vi "pulsed ODMR.vi"() -> ()   [LabVIEW 2012]
uses:
  <vilib>/DAQmx/read.llb/DAQmx Read (Counter U32 1Chan 1Samp).vi
  <vilib>/Utility/file.llb/Write To Spreadsheet File (DBL).vi
  <vilib>/DAQmx/miscellaneous.llb/DAQmx Fill In Error Info.vi
  <vilib>/DAQmx/create/channels.llb/DAQmx Create Channel (CI-Count Edges).vi
  <vilib>/DAQmx/create/channels.llb/DAQmx Create Channel (CO-Pulse Generation-Ticks).vi
  <vilib>/DAQmx/configure/timing.llb/DAQmx Timing (Implicit).vi
  <vilib>/DAQmx/configure/timing.llb/DAQmx Timing (Sample Clock).vi
  <resource>/objmgr/daqmx.rc
panel:
  out "Scan":i32=1
  in  "N Scans":i32=200
  out "freq":dbl=3169000000.0
  out "diff":dbl=864.0
  out "loop":i32=169
  in  "file path (dialog if empty)":path=path "C:/Users/Ouyang Group/Documents/Data/10-10-16/MNP 4 on CPW 5mW x157 y142 B0.4V pulsed ODMR sweep 2"
  out "Z Position 2":dbl=37.2
  out "Y Position 2":dbl=132.5360878371843
  out "X Position 2":dbl=154.08405055143967
  in  "CW for tracking":bool
  in  "Y Parameters":T1={"Number of Y Steps"=200, "Max Y (V)"=2.0, "Min Y (V)"=-2.0}
  in  "X":T2={"Number of X Steps"=200, "Max X (V)"=2.0, "Min X (V)"=-2.0}
  in  "Z Position":dbl=37.2
  in  "Y Position":dbl=132.0
  in  "X Position":dbl=154.0
  in  "Z-track?":bool=TRUE
  out "XY Graph":cluster{"Y":dbl[], "Y":dbl[]}[](graph)=[{"Y"=[3000000000.0, 3001000000.0, 3002000000.0, 3003000000.0, 3004000000.0, 3005000000.0, 3006000000.0, 3007000000.0, 3008000000.0, 3009000000.0, 3010000000.0, 3011000000.0, 3012000000.0, 3013000000.0, 3014000000.0, 3015000000.0, 3016000000.0, 3017000000.0, 3018000000.0, 3019000000.0, 3020000000.0, 3021000000.0, 3022000000.0, 3023000000.0, 3024000000.0, 3025000000.0, 3026000000.0, 3027000000.0, 3028000000.0, 3029000000.0, 3030000000.0, 3031000000.0, 3032000000.0, 3033000000.0, 3034000000.0, 3035000000.0, 3036000000.0, 3037000000.0, 3038000000.0, 3039000000.0, 3040000000.0, 3041000000.0, 3042000000.0, 3043000000.0, 3044000000.0, 3045000000.0, 3046000000.0, 3047000000.0, 3048000000.0, 3049000000.0, 3050000000.0, 3051000000.0, 3052000000.0, 3053000000.0, 3054000000.0, 3055000000.0, 3056000000.0, 3057000000.0, 3058000000.0, 3059000000.0, 3060000000.0, 3061000000.0, 3062000000.0, 3063000000.0, 3064000000.0, 3065000000.0, 3066000000.0, 3067000000.0, 3068000000.0, 3069000000.0, 3070000000.0, 3071000000.0, 3072000000.0, 3073000000.0, 3074000000.0, 3075000000.0, 3076000000.0, 3077000000.0, 3078000000.0, 3079000000.0, 3080000000.0, 3081000000.0, 3082000000.0, 3083000000.0, 3084000000.0, 3085000000.0, 3086000000.0, 3087000000.0, 3088000000.0, 3089000000.0, 3090000000.0, 3091000000.0, 3092000000.0, 3093000000.0, 3094000000.0, 3095000000.0, 3096000000.0, 3097000000.0, 3098000000.0, 3099000000.0, 3100000000.0, 3101000000.0, 3102000000.0, 3103000000.0, 3104000000.0, 3105000000.0, 3106000000.0, 3107000000.0, 3108000000.0, 3109000000.0, 3110000000.0, 3111000000.0, 3112000000.0, 3113000000.0, 3114000000.0, 3115000000.0, 3116000000.0, 3117000000.0, 3118000000.0, 3119000000.0, 3120000000.0, 3121000000.0, 3122000000.0, 3123000000.0, 3124000000.0, 3125000000.0, 3126000000.0, 3127000000.0, 3128000000.0, 3129000000.0, 3130000000.0, 3131000000.0, 3132000000.0, 3133000000.0, 3134000000.0, 3135000000.0, 3136000000.0, 3137000000.0, 3138000000.0, 3139000000.0, 3140000000.0, 3141000000.0, 3142000000.0, 3143000000.0, 3144000000.0, 3145000000.0, 3146000000.0, 3147000000.0, 3148000000.0, 3149000000.0, 3150000000.0, 3151000000.0, 3152000000.0, 3153000000.0, 3154000000.0, 3155000000.0, 3156000000.0, 3157000000.0, 3158000000.0, 3159000000.0, 3160000000.0, 3161000000.0, 3162000000.0, 3163000000.0, 3164000000.0, 3165000000.0, 3166000000.0, 3167000000.0, 3168000000.0, 3169000000.0], "Y"=[20897.0, 22852.0, 22779.0, 22894.0, 22927.0, 22741.0, 22573.0, 22733.0, 22830.0, 22883.0, 22762.0, 22899.0, 22761.0, 22773.0, 22842.0, 22907.0, 22850.0, 22605.0, 22781.0, 22681.0, 22700.0, 22960.0, 23015.0, 22551.0, 22696.0, 22371.0, 22868.0, 22865.0, 22767.0, 22787.0, 22656.0, 22872.0, 22848.0, 22750.0, 22901.0, 22775.0, 22816.0, 21819.0, 22361.0, 22464.0, 22800.0, 22880.0, 22472.0, 22759.0, 22543.0, 22595.0, 23074.0, 22794.0, 22857.0, 22851.0, 22603.0, 22581.0, 22045.0, 22687.0, 22517.0, 22600.0, 22685.0, 22887.0, 22876.0, 22789.0, 22503.0, 22751.0, 22684.0, 22564.0, 22897.0, 22744.0, 21980.0, 22771.0, 22841.0, 22311.0, 22234.0, 22304.0, 22403.0, 22585.0, 22374.0, 22604.0, 22287.0, 22575.0, 22599.0, 22689.0, 22662.0, 22060.0, 22437.0, 22293.0, 21954.0, 21800.0, 21174.0, 20810.0, 20547.0, 20230.0, 20049.0, 19600.0, 19389.0, 18817.0, 18827.0, 18800.0, 18771.0, 19210.0, 19068.0, 19533.0, 19442.0, 19668.0, 19746.0, 20480.0, 21116.0, 21287.0, 21615.0, 21711.0, 21860.0, 22239.0, 22301.0, 22345.0, 22646.0, 22502.0, 22803.0, 22744.0, 22476.0, 22049.0, 22378.0, 22415.0, 22489.0, 22623.0, 22255.0, 22383.0, 22791.0, 22426.0, 22564.0, 22666.0, 22587.0, 22692.0, 22619.0, 22746.0, 22870.0, 22967.0, 22739.0, 23010.0, 22733.0, 22399.0, 22777.0, 22571.0, 22573.0, 22914.0, 22383.0, 23082.0, 22534.0, 22649.0, 22510.0, 22903.0, 22967.0, 22609.0, 22872.0, 22608.0, 22798.0, 22757.0, 22774.0, 22548.0, 22722.0, 22710.0, 22449.0, 22814.0, 22959.0, 22831.0, 22570.0, 22918.0, 23017.0, 22810.0, 22802.0, 22761.0, 22627.0, 22371.0]}]
  in  "Freq Max":dbl=3120000000.0
  in  "Freq  Step":dbl=250000000.0
  in  "Freq Min":dbl=3060000000.0
  in  "power":dbl=-9.0
  in  "stop":bool
  in  "Path to spinapi.dll":path=path "C:/SpinCore/SpinAPI/dll/spinapi64.dll"
  in  "Pulse offset":dbl
  in  "Rabi Freq":dbl=8895000.0
  in  "MW Delay":dbl=2e-08
  in  "APD signal width":dbl=3e-07
  in  "Signal Delay":dbl=7.6e-07
  in  "AOM Rest time":dbl=1e-06
  in  "AOM Pulse length":dbl=2.5e-06
  in  "N Loop":i32=100000
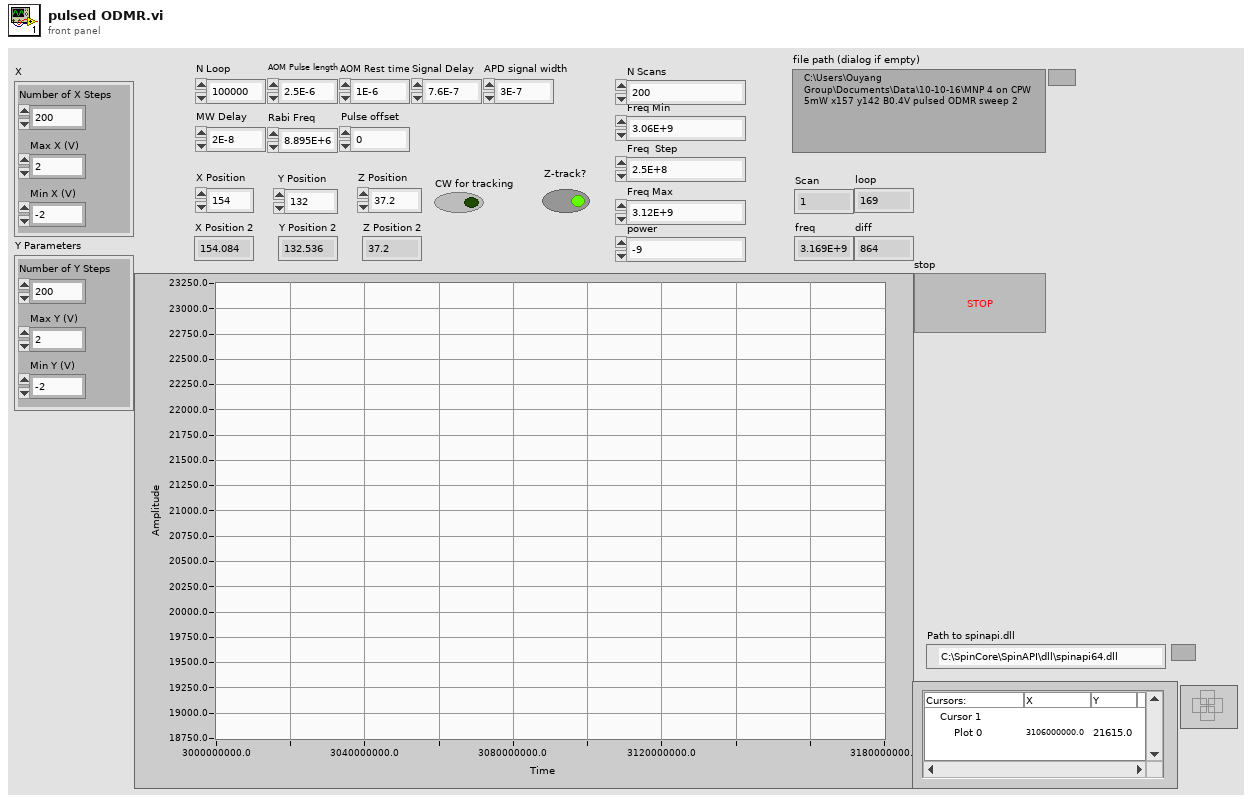
[diagram p1: front panel]
types:
  T1 = cluster{"Number of Y Steps":i32, "Max Y (V)":dbl, "Min Y (V)":dbl}
  T2 = cluster{"Number of X Steps":i32, "Max X (V)":dbl, "Min X (V)":dbl}
  T3 = enum16{"Pulse Program", "Frequency Registers", "TX Phase Registers", "RX Phase Registers"}
  T4 = cluster{"Instruct Data":i32, "Op Code":i32, "Flags":bool[], "Comments":string, "Time (s)":dbl}[]
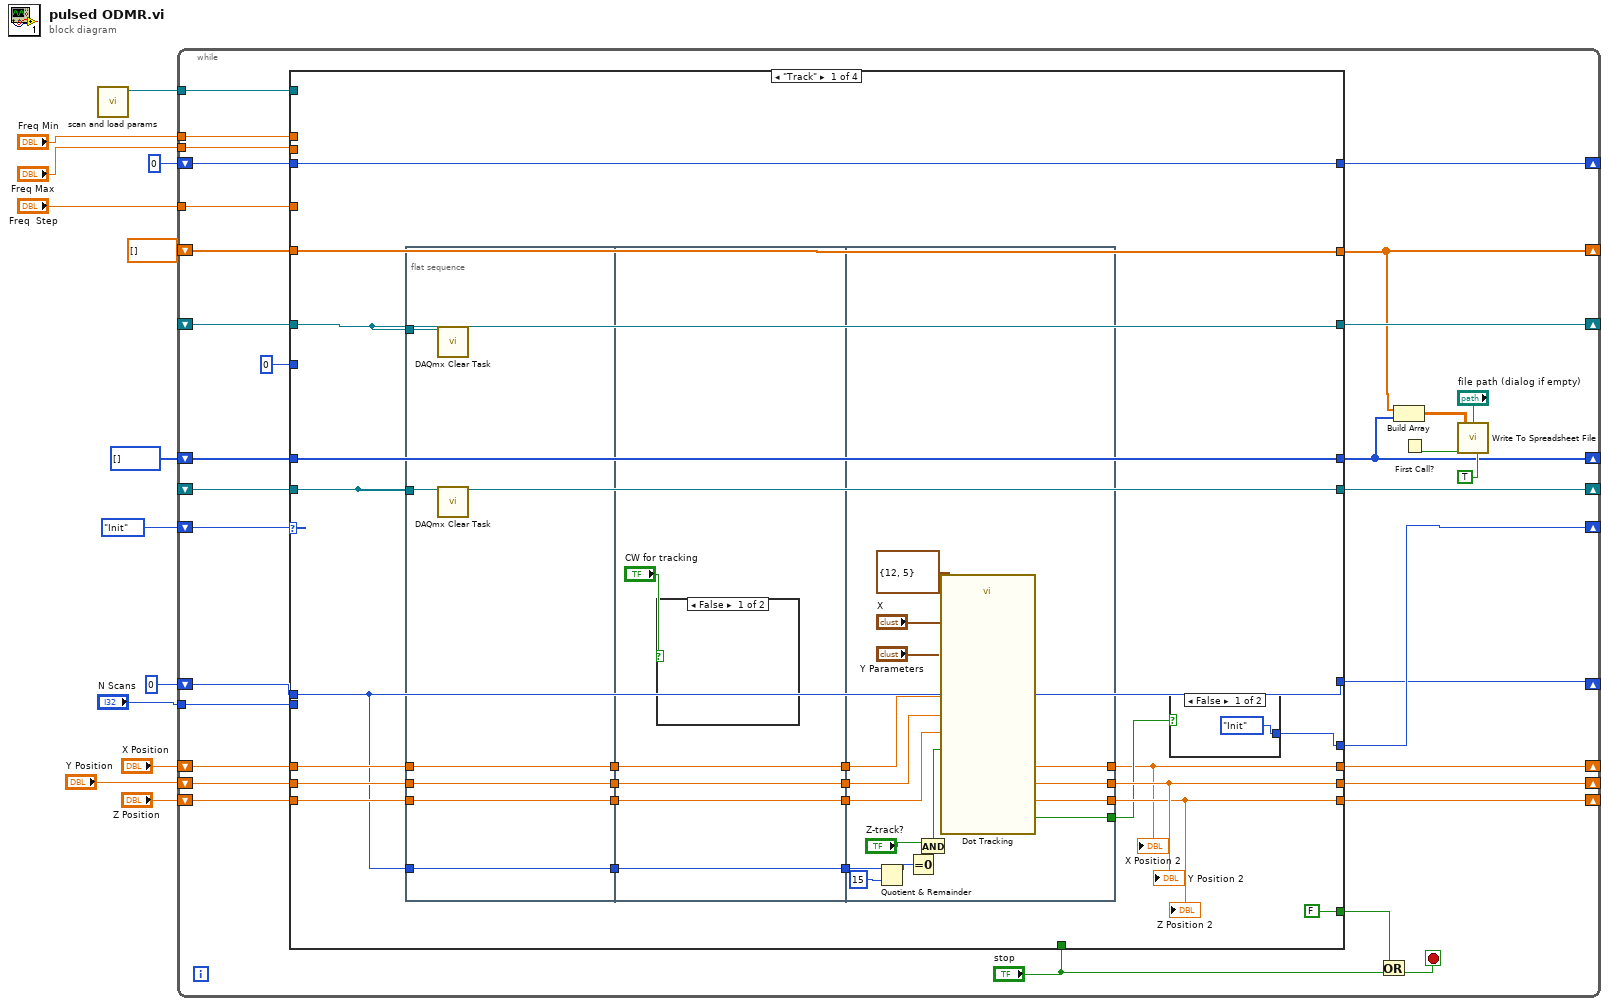
[diagram p0: block diagram]
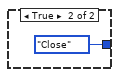
[diagram p2: hidden frame]
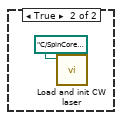
[diagram p3: hidden frame]
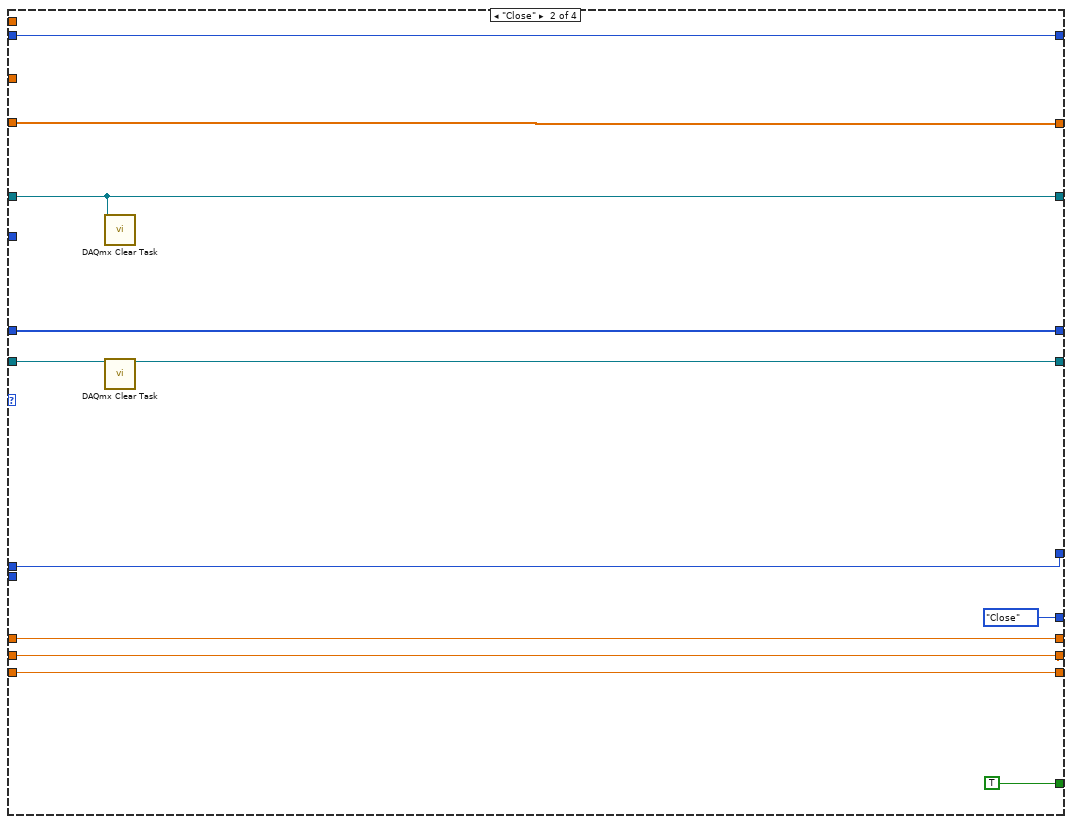
[diagram p4: hidden frame]
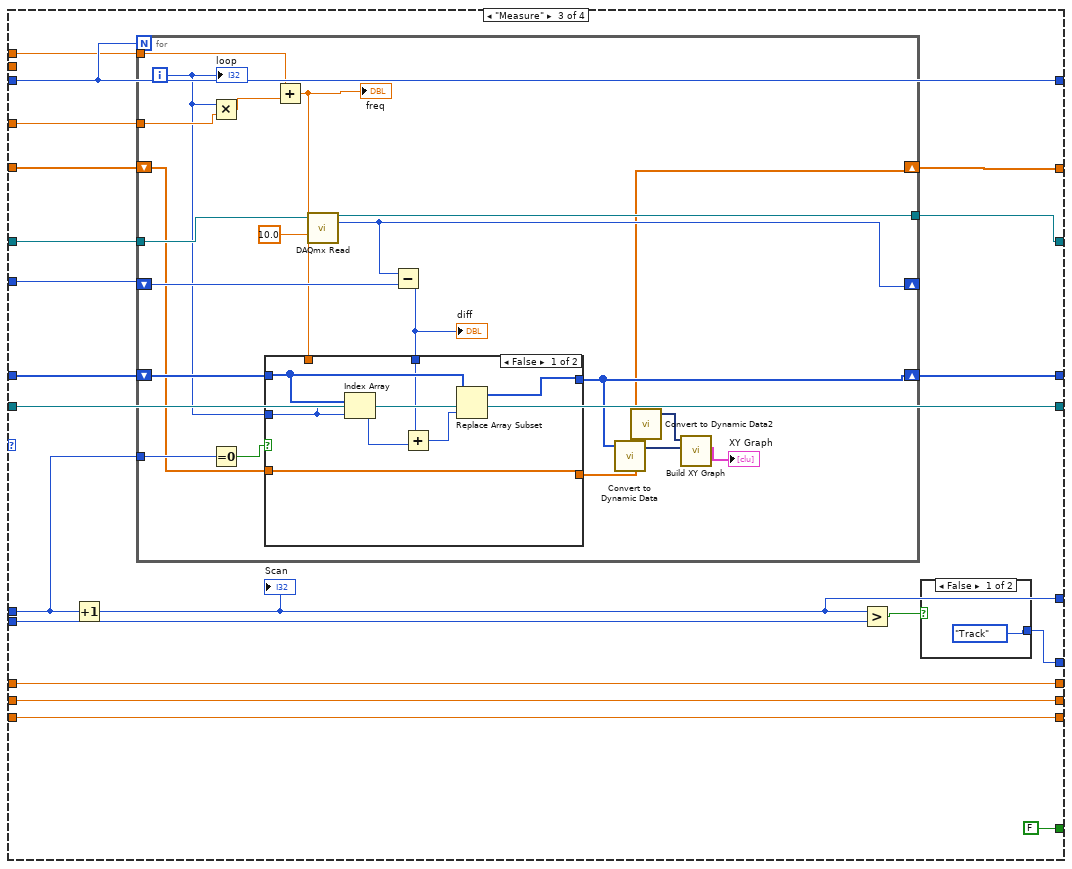
[diagram p5: hidden frame]
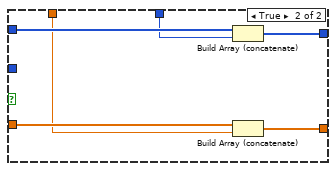
[diagram p6: hidden frame]
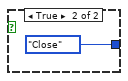
[diagram p7: hidden frame]
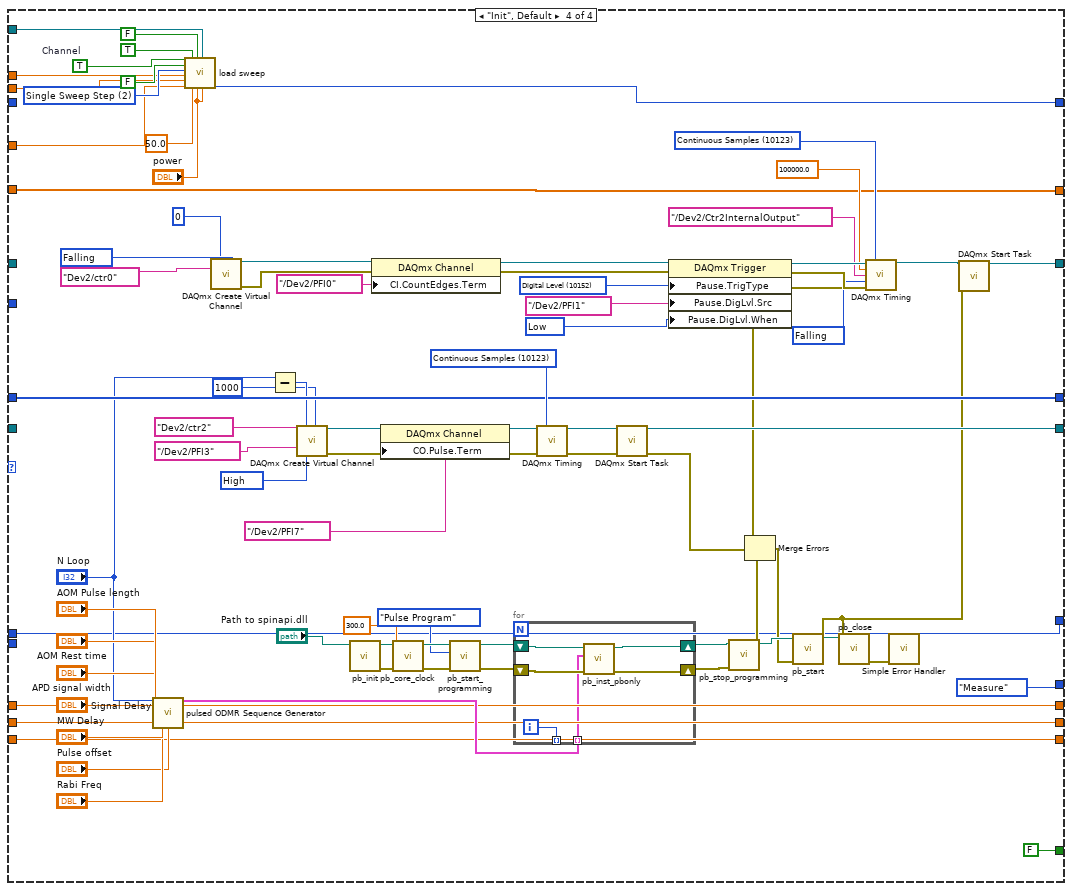
[diagram p8: hidden frame]
diagram:
  n1 = call "scan and load params.vi"() -> ("Serial Port Select"=w7:refnum<visa-resource-name>)  [unwired: 9 out]
  n2 = while {
    shift-right: [w40] -> _
    shift-left: enum16{"Init", "Track", "Measure", "Close", ""}."Init" -> [w46]
    shift-right: [w45] -> _
    shift-left: _ -> [w33]
    shift-right: [w44] -> _
    shift-left: _ -> [w34]
    shift-right: [w15] -> _
    shift-left: u32[] [] -> [w42]
    shift-right: [w28] -> _
    shift-left: dbl[] [] -> [w41]
    shift-right: [w39] -> _
    shift-left: "X Position" -> [w30]
    shift-right: [w38] -> _
    shift-left: "Y Position" -> [w36]
    shift-right: [w37] -> _
    shift-left: "Z Position" -> [w35]
    tunnel: w7 -> [w23]
    tunnel: "Freq  Step" -> [w20]
    tunnel: "Freq Max" -> [w21]
    tunnel: "Freq Min" -> [w22]
    shift-right: [w19] -> _
    shift-left: u16 0 ("Number\nof Points") -> [w18]
    tunnel: "N Scans" -> [w17]
    shift-right: [w14] -> _
    shift-left: 0 -> [w16]
    stop <- w32 stop-if-true
    n3 = case shown="\"Track\"" w46 {
      tunnel: [w53 w110 w124 w195] -> w45
      tunnel: [w52 w109 w117 w194] -> w44
      tunnel: "stop" -> [_ _ _ _]
      tunnel: w42 -> [w62 w108 w130 w192]
      tunnel: w41 -> [w57 w103 w129 w188]
      tunnel: [w62 w108 w128 w192] -> w15
      tunnel: [w57 w103 w121 w188] -> w28
      tunnel: [w61 enum16{"Init", "Track", "Measure", "Close", ""}."Close" w127 enum16{"Init", "Track", "Measure", "Close", ""}."Measure"] -> w40
      tunnel: [w50 w102 w120 w187] -> w39
      tunnel: [w69 w107 w123 w190] -> w38
      tunnel: [w68 w106 w122 w189] -> w37
      tunnel: w36 -> [w65 w107 w123 w190]
      tunnel: w35 -> [w63 w106 w122 w189]
      tunnel: w34 -> [w52 w109 w125 _]
      tunnel: w33 -> [w53 w110 w124 _]
      tunnel: [FALSE TRUE FALSE FALSE] -> w31
      tunnel: w30 -> [w58 w102 w120 w187]
      tunnel: u32 0 ("data") -> [_ _ w119 _]
      tunnel: w23 -> [_ _ _ w180]
      tunnel: w22 -> [_ _ w116 w172]
      tunnel: w21 -> [_ _ _ w171]
      tunnel: w20 -> [_ _ w115 w170]
      tunnel: [w51 w101 w118 w169] -> w19
      tunnel: w18 -> [w51 w101 w118 _]
      tunnel: w17 -> [_ _ w113 _]
      tunnel: w16 -> [w47 w100 w111 w168]
      tunnel: [w47 w100 w112 w168] -> w14
      frame "Track" {
        n4 = flat-sequence {
          tunnel: w63 -> [w75]
          tunnel: w65 -> [w76]
          tunnel: w58 -> [w77]
          tunnel: [w77] -> w56
          tunnel: [w76] -> w55
          tunnel: [w75] -> w54
          tunnel: w53 -> [w74]
          tunnel: w52 -> [w73]
          tunnel: [w72] -> w48
          tunnel: w47 -> [w72]
          tunnel: [w82] -> w67
          tunnel: [w81] -> w66
          tunnel: [w80] -> w64
          tunnel: w56 -> [w82]
          tunnel: w55 -> [w81]
          tunnel: w54 -> [w80]
          tunnel: [w78] -> w49
          tunnel: w48 -> [w78]
          tunnel: [w99] -> w50
          tunnel: [w98] -> w69
          tunnel: [w97] -> w68
          tunnel: w67 -> [w96]
          tunnel: w66 -> [w95]
          tunnel: w64 -> [w94]
          tunnel: [w90] -> w60
          tunnel: w49 -> [w84]
          frame #0 {
            n5 = call <vilib>:"DAQmx Clear Task.vi"("task in"=w73) -> ()  [unwired: 14 in, 1 out]
            n6 = call <vilib>:"DAQmx Clear Task.vi"("task in"=w74) -> ()  [unwired: 14 in, 1 out]
          }
          frame #1 {
            n7 = case shown="False" "CW for tracking" {
              frame False {
              }
              frame True {
                n8 = call "Load and init CW laser.vi"("path in"=path "C:/SpinCore/SpinAPI/dll/spinapi64.dll") -> ()  [unwired: 11 in]
              }
            }
          }
          frame #2 {
            n9 = Quotient & Remainder(x=w84, y=15) -> (x-y*floor(x/y)=w88:i32)  [unwired: 1 out]
            n10 = Equal To 0?(x=w88) -> (x = 0?=w87:bool)
            n11 = And(x="Z-track?", y=w87) -> (x .and. y?=w85:bool)
            n12 = call "Dot Tracking.vi"("X"="X", "Y Parameters"="Y Parameters", "RS232 settings"=cluster{"Portnumber":i32, "Baudrate":u16} {"Portnumber"=12, "Baudrate"=5}, "X Pos"=w96, "Y pos"=w95, "Z Pos"=w94, "Z-track?"=w85) -> ("X Position"=w99:dbl, "Y Position"=w98:dbl, "Z Position"=w97:dbl, "Gave up?"=w90:bool)  [unwired: 2 in, 3 out]
          }
        }
        n13 = case shown="False" w60 {
          tunnel: [enum16{"Init", "Track", "Measure", "Close", ""}."Init" enum16{"Init", "Track", "Measure", "Close", ""}."Close"] -> w61
          frame False {
          }
          frame True {
          }
        }
        "X Position 2" <- w50
        "Y Position 2" <- w69
        "Z Position 2" <- w68
      }
      frame "Close" {
        n14 = call <vilib>:"DAQmx Clear Task.vi"("task in"=w109) -> ()  [unwired: 14 in, 1 out]
        n15 = call <vilib>:"DAQmx Clear Task.vi"("task in"=w110) -> ()  [unwired: 14 in, 1 out]
      }
      frame "Measure" {
        n16 = Increment(x=w111) -> (x+1=w112:i32)
        "Scan" <- w112
        n17 = for {
          N: w118 -> [_]
          shift-right: [w141] -> w128
          shift-left: w130 -> [w142]
          shift-right: [w132] -> w121
          shift-left: w129 -> [w133]
          tunnel: w125 -> [w149]
          shift-right: [w144] -> _
          shift-left: w119 -> [w146]
          tunnel: [w145] -> w117
          tunnel: w116 -> [w140]
          tunnel: w115 -> [w139]
          tunnel: w111 -> [w136]
          i -> [w134]
          n18 = Multiply(x=w134, y=w139) -> (x*y=w138:dbl)
          n19 = Equal To 0?(x=w136) -> (x = 0?=w135:bool)
          n20 = Add(x=w140, y=w138) -> (x+y=w131:dbl)
          "freq" <- w131
          n21 = call-poly <vilib>:"DAQmx Read.vi"("task/channels in"=w149, "timeout"=10.0) -> ("task out"=w145:refnum<k21>, "data"=w144:u32)  [unwired: 11 in, 1 out]
          n22 = Subtract(x=w144, y=w146) -> (x-y=w137:u32)
          "diff" <- w137
          n23 = case shown="False" w135 {
            tunnel: w142 -> [w157 w163]
            tunnel: [w152 w162] -> w141
            tunnel: w137 -> [w154 w161]
            tunnel: w134 -> [w156 _]
            tunnel: w133 -> [w151 w160]
            tunnel: [w151 w159] -> w132
            tunnel: w131 -> [_ w158]
            frame False {
              n24 = Index Array(array=w157, index=w156) -> (element=w155:u32)
              n25 = Add(x=w154, y=w155) -> (x+y=w153:u32)
              n26 = Replace Array Subset(array=w157, new element=w153, index=w156) -> (w152:u32[])
            }
            frame True {
              n27 = Build Array (concatenate)(w163, w161) -> (w162:u32[])
              n28 = Build Array (concatenate)(w160, w158) -> (w159:dbl[])
            }
          }
          n29 = call "Convert to Dynamic Data"("Array"=w141) -> ("Dynamic Data Type"=w147:dynamicdata)  [unwired: 3 in]
          n30 = call "Convert to Dynamic Data2"("Array"=w132) -> ("Dynamic Data Type"=w148:dynamicdata)  [unwired: 3 in]
          n31 = call "Build XY Graph"("Y Input"=w147, "X Input"=w148) -> ("XY Graph"=→"XY Graph":cluster{"Y":dbl[], "Y":dbl[]}[])  [unwired: 3 in, 6 out]
          "loop" <- w134
        }
        n32 = Greater?(x=w112, y=w113) -> (0:w114:bool)
        n33 = case shown="False" w114 {
          tunnel: [enum16{"Init", "Track", "Measure", "Close", ""}."Track" enum16{"Init", "Track", "Measure", "Close", ""}."Close"] -> w127
          frame False {
          }
          frame True {
          }
        }
      }
      frame "Init", Default {
        w166 = 10171 items=["Rising"=10280, "Falling"=10171] ("active edge")
        w167 = 10192 items=["High"=10192, "Low"=10214] ("idle state")
        w175 = 2 items=["No Triggers", "Full Frequency Sweep", "Single Sweep Step", "Stop All", "Digital RF On/Off", "Remove Interrupts", "Reserved 1", "Reserved 2", "Ext AM Modulation", "Ext FM Modulation"] ("Trigger")
        w177 = TRUE  # Channel
        w181 = 1000 ("y")
        w203 = 10123 items=["Finite Samples"=10178, "Continuous Samples"=10123, "Hardware Timed Single Point"=12522] ("sample mode")
        w221 = 10214 items=["High"=10192, "Low"=10214] ("Pause.DigLvl.When")
        w223 = 10152 items=["Analog Level"=10101, "Analog Window"=10103, "Digital Level"=10152, "Digital Pattern"=10398, "None"=10230] ("Pause.TrigType")
        w210 = 10123 items=["Finite Samples"=10178, "Continuous Samples"=10123, "Hardware Timed Single Point"=12522] ("sample mode")
        w199 = 10171 items=["Rising"=10280, "Falling"=10171] ("edge")
        n34 = call "pulsed ODMR Sequence Generator.vi"("N Loop"="N Loop", "Rabi Frequency"="Rabi Freq", "AOM Pulse length"="AOM Pulse length", "AOM Rest time"="AOM Rest time", "Signal Delay"="Signal Delay", "APD signal width"="APD signal width", "MW Delay"="MW Delay", "Pulse offset"="Pulse offset") -> ("Pulse Sequence"=w224:T4)  [unwired: 7 in]
        n35 = call "load sweep.vi"("Channel"=w177, "Sweep\nContinuously"=FALSE ("Sweep\nContinuously"), "Trigger"=w175, "Start Frequency"=w172, "Stop Frequency"=w171, "Step Size MHz"=w170, "RF On"=TRUE, "Step Time (mS)"=50.0, "load?"=FALSE, "Start Amplitude"="power", "Serial Port Select"=w180, "Stop Amplitude"="power") -> ("Number\nof Points"=w169:u16)  [unwired: 7 in]
        n36 = call-poly <vilib>:"DAQmx Create Virtual Channel.vi"("initial count"=u32 0, "edge"=w199, "counter"=tag "Dev2/ctr0") -> ("task out"=w219:refnum<k21>, "error out"=w216:errorcluster)  [unwired: 6 in, 5 out]
        n37 = Subtract(x="N Loop", y=w181) -> (x-y=w183:i32)
        n38 = call-poly <vilib>:"DAQmx Create Virtual Channel.vi"("high ticks"=w183, "low ticks"=w181, "counter"=tag "Dev2/ctr2", "source of ticks"=tag "/Dev2/PFI3" ("source"), "idle state"=w167) -> ("task out"=w207:refnum<k21>, "error out"=w205:errorcluster)  [unwired: 9 in]
        n39 = call "pb_init.vi"("path in"="Path to spinapi.dll") -> ("error out"=w230:errorcluster, "path out"=w228:path)  [unwired: 3 in, 6 out]
        n40 = property class="DAQmx Channel"(reference=w219, error in=w216, "CI.CountEdges.Term"=tag "/Dev2/PFI0") -> (reference out=w220:refnum<k21>, error out=w218:errorcluster)
        n41 = property class="DAQmx Channel"(reference=w207, "CO.Pulse.Term"=tag "/Dev2/PFI7") -> (reference out=w202:refnum<k21>)  [unwired: 1 in, 1 out]
        n42 = call "pb_core_clock.vi"("error in (no error)"=w230, "clock_freq (MHz)"=300.0, "path in"=w228) -> ("error out"=w231:errorcluster, "path out"=w229:path)  [unwired: 7 in]
        n43 = call "pb_start_programming.vi"("error in (no error)"=w231, "Device"=T3."Pulse Program", "path in"=w229) -> ("error out"=w234:errorcluster, "path out"=w233:path)  [unwired: 1 in, 6 out]
        n44 = for {
          shift-right: [w249] -> w235
          shift-left: w233 -> [w251]
          shift-right: [w248] -> w236
          shift-left: w234 -> [w250]
          tunnel: [w247] -> _ mode=indexing
          tunnel: w224 -> [w246] mode=indexing
          i -> [w247]
          n45 = call "pb_inst_pbonly.vi"("error in (no error)"=w250, "PB Instruction"=w246, "path in"=w251) -> ("error out"=w248:errorcluster, "path out"=w249:path)  [unwired: 2 in, 5 out]
        }
        n46 = call-poly <vilib>:"DAQmx Timing.vi"("task/channels in"=w202, "sample mode"=w203, "error in"=w205) -> ("task out"=w206:refnum<k21>, "error out"=w204:errorcluster)  [unwired: 11 in]
        n47 = call <vilib>:"DAQmx Start Task.vi"("task/channels in"=w206, "error in"=w204) -> ("task out"=w195:refnum<k21>, "error out"=w198:errorcluster)  [unwired: 12 in]
        n48 = property class="DAQmx Trigger"(reference=w220, error in=w218, "Pause.TrigType"=w223, "Pause.DigLvl.Src"=tag "/Dev2/PFI1", "Pause.DigLvl.When"=w221) -> (reference out=w215:refnum<k21>, error out=w214:errorcluster)
        n49 = call "pb_stop_programming.vi"("error in (no error)"=w236, "path in"=w235) -> ("error out"=w196:errorcluster, "path out"=w226:path)  [unwired: 1 in, 7 out]
        n50 = call-poly <vilib>:"DAQmx Timing.vi"("task/channels in"=w215, "sample mode"=w210, "rate"=100000.0, "source"=tag "/Dev2/Ctr2InternalOutput", "active edge"=w166, "error in"=w214) -> ("task out"=w212:refnum<k21>, "error out"=w185:errorcluster)  [unwired: 8 in]
        n51 = Merge Errors(w185, w198, w196) -> (w197:errorcluster)
        n52 = call "pb_start.vi"("error in (no error)"=w197, "path in"=w226) -> ("error out"=w184:errorcluster, "path out"=w225:path)  [unwired: 1 in, 7 out]
        n53 = call "pb_close.vi"("error in (no error)"=w184, "path in"=w225) -> ("error out"=w238:errorcluster)  [unwired: 9 out]
        n54 = call <vilib>:"Simple Error Handler.vi"("error in (no error)"=w238) -> ()  [unwired: 1 in, 8 out]
        n55 = call <vilib>:"DAQmx Start Task.vi"("task/channels in"=w212, "error in"=w184) -> ("task out"=w194:refnum<k21>)  [unwired: 13 out]
      }
    }
    n56 = Or(x=w31, y="stop") -> (x .or. y?=w32:bool)
    n57 = Build Array(w28, w15) -> (w27:dbl[][])
    n58 = First Call?() -> (First Call?: T/F=w24:bool)
    n59 = call-poly <vilib>:"Write To Spreadsheet File.vi"("transpose? (no:F)"=TRUE, "append to file? (new file:F)"=w24, "2D data"=w27, "file path (dialog if empty)"="file path (dialog if empty)") -> ()  [unwired: 4 in, 1 out]
  }
